vi "SetTypedConfiguration.vi"(6 "private? (F)":bool, 8 "error in (no error)":errorcluster, 9 "Name (empty: value name)":string, 10 "Default value":variant, 11 "SMO":refnum<class "SMO.lvclass">) -> (0 "error out":errorcluster, 2 "keys written":string[](array[string]), 3 "SMO out":refnum<class "SMO.lvclass">)   [LabVIEW 2013, in "SMO.lvclass"]
uses:
  SMO.lvclass
  Support/Attribute.Config/Attribute.Config.lvclass/Attribute.Config.ctl
  <vilib>/LabVIEW Open Source/Configuration Manager/Manager/ConfigManager.lvclass
  <vilib>/LabVIEW Open Source/Configuration Manager/Manager/ConfigManager.lvclass/ConfigManager.ctl
  <vilib>/LabVIEW Open Source/Configuration Manager/Serializer/Serializer.lvclass
  <vilib>/LabVIEW Open Source/Configuration Manager/Encoding/Encoding.lvclass
  <vilib>/LabVIEW Open Source/Configuration Manager/Encryption/Encryption.lvclass
  <vilib>/LabVIEW Open Source/Configuration Manager/Manager/Write.vi
  <vilib>/LabVIEW Open Source/Configuration Manager/Manager/Read Serializer.vi
  <vilib>/LabVIEW Open Source/Configuration Manager/Manager/Read Encoding.vi
  <vilib>/LabVIEW Open Source/Configuration Manager/Manager/Read Encryption.vi
  <vilib>/LabVIEW Open Source/Configuration Manager/Manager/Decompose KVPs.vi
  <vilib>/Utility/VariantDataType/GetTypeInfo.vi
  Support/Attribute.Config/Attribute.Config.lvclass
panel:
  # "For instructions on how to use the JKI State Machine Objects, examples and video tutorials, visit:\nhttp://jki.net/state-machine-objects/\n\nJKI State Machine Objects™\nhttp://jki.net/state-machine-objects/\nCopyright (C) 2005-2015, JKI <info@jki.net>\nALL RIGHTS RESERVED"
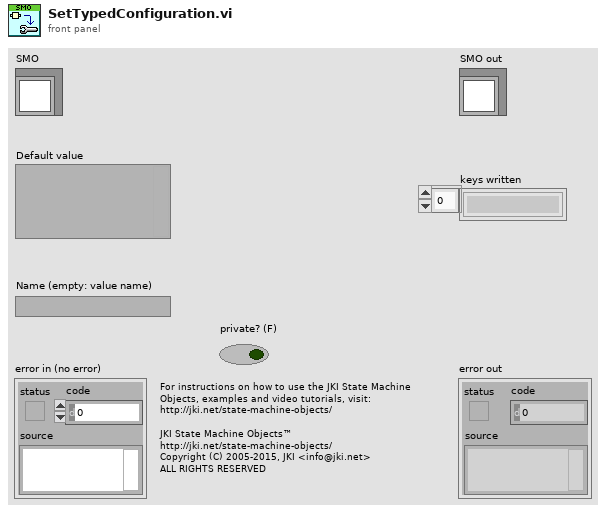
[diagram p1: front panel]
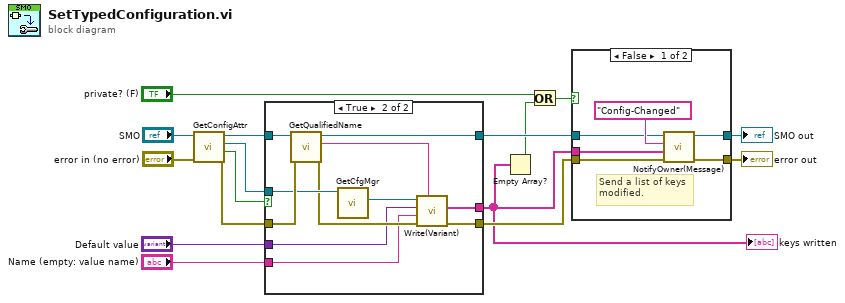
[diagram p0: block diagram]
diagram:
  n1 = call "GetConfigAttr.vi"("error in (no error)"="error in (no error)", "SMO in"="SMO") -> ("error out"=w11:errorcluster, "found"=w13:bool, "Attribute.Config"=w12:refnum<class "Attribute.Config.lvclass">, "SMO out"=w14:refnum<class "SMO.lvclass">)  [unwired: 6 in]
  n2 = case shown="True" w13 {
    tunnel: w12 -> [_ w26]
    tunnel: w14 -> [w18 w29]
    tunnel: [w18 w28] -> w6
    tunnel: w11 -> [w17 w27]
    tunnel: [w17 w23] -> w5
    tunnel: "Default value" -> [_ w21]
    tunnel: "Name (empty: value name)" -> [_ w20]
    tunnel: [_ w24] -> w1
    frame False {
    }
    frame True {
      n3 = call "GetQualifiedName.vi"("error in (no error)"=w27, "SMO"=w29) -> ("error out"=w22:errorcluster, "Qualified Name"=w19:string, "SMO out"=w28:refnum<class "SMO.lvclass">)  [unwired: 7 in]
      n4 = call "GetCfgMgr.vi"("Attribute.Config in"=w26) -> ("CfgMgr"=w25:refnum<class "ConfigManager.lvclass">)  [unwired: 9 in, 1 out]
      n5 = call <vilib>:"Write(Variant).vi"("Qualified Name"=w19, "error in (no error)"=w22, "Name (empty: va;ue name)"=w20, "value"=w21, "ConfigManager in"=w25) -> ("error out"=w23:errorcluster, "keys written"=w24:string[])  [unwired: 4 in, 1 out]
    }
  }
  "keys written" <- w1
  n6 = Empty Array?(array=w1) -> (empty?=w4:bool)
  n7 = Or(x="private? (F)", y=w4) -> (x .or. y?=w2:bool)
  n8 = case shown="False" w2 {
    tunnel: w6 -> [w34 w37]
    tunnel: [w33 w37] -> w16
    tunnel: w5 -> [w32 w36]
    tunnel: [w31 w36] -> w15
    tunnel: w1 -> [w30 _]
    frame False {
      # "Send a list of keys\nmodified."
      n9 = call "NotifyOwner(Message).vi"("error in (no error)"=w32, "Payload"=w30, "Message (empty : payload label)"="Config-Changed", "SMO in"=w34) -> ("error out"=w31:errorcluster, "SMO out"=w33:refnum<class "SMO.lvclass">)  [unwired: 6 in]
    }
    frame True {
      # "No notification change\nevent to caller on\nprivate config change"
    }
  }
  "error out" <- w15
  "SMO out" <- w16
